vi "PXI Clear Counter Task.vi"(2 "error in":errorcluster) -> (0 "error out":errorcluster)   [LabVIEW 2015]
uses:
  PXI Globals.vi
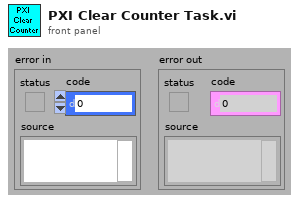
[diagram p1: front panel]
types:
  T1 = typedef "Task Struct.ctl" = cluster{"Task name":string, "Task":refnum<k21>, "Dual-channel task?":bool, "Regenerate?":bool, "Clear?":bool}
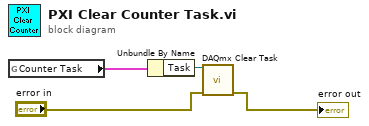
[diagram p0: block diagram]
diagram:
  n1 = global read "PXI Globals.vi" "Counter Task"() -> (w4:T1)
  n2 = Unbundle By Name(w4) -> ("Task"=w1:refnum<k21>)
  n3 = call <vilib>:"DAQmx Clear Task.vi"("task in"=w1, "error in"="error in") -> ("error out"=→"error out":errorcluster)  [unwired: 13 in]
